vi "StatusUpdateByModID.vi"(8 "error in (no error)":errorcluster, 10 "Status":string, 11 "Accessors:Module ID":i32) -> (0 "error out":errorcluster)   [LabVIEW 2018, in "SensorPlugins.lvlib"]
uses:
  SensorPlugins.lvlib
  SensorShared/clEventType.ctl
  SensorShared/SensorShared.lvlib
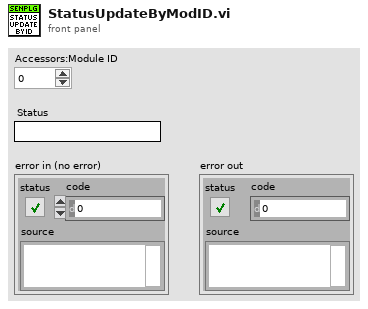
[diagram p1: front panel]
types:
  T1 = typedef "SensorShared.lvlib/clEventType.ctl" = cluster{"ModuleID":i32, "Data":variant}
  T2 = typedef "SensorShared.lvlib/clBroadcastEvents.ctl" = cluster{"DidInit":refnum<user-event>, "StatusUpdate":refnum<user-event>, "ErrorReport":refnum<user-event>, "DidStop":refnum<user-event>, "PathToINI":refnum<user-event>, "SensorReport":refnum<user-event>, "SensorConfig":refnum<user-event>}
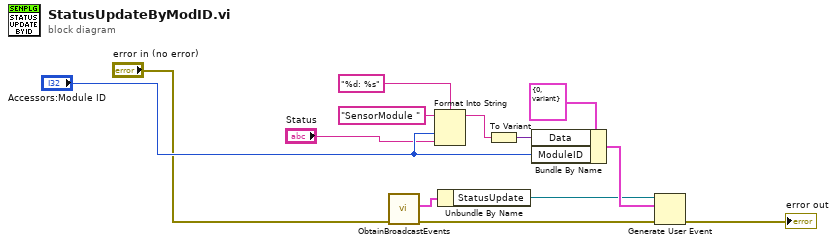
[diagram p0: block diagram]
diagram:
  n1 = call "ObtainBroadcastEvents.vi"("error in (no error)"="error in (no error)") -> ("error out"=w11:errorcluster, "clBroadcastEvents"=w1:T2)  [unwired: 9 in]
  n2 = Format Into String(format string="%d: %s", initial string="SensorModule ", "Accessors:Module ID", "Status") -> (resulting string=w8:string)  [unwired: 1 in, 1 out]
  n3 = Unbundle By Name(w1) -> ("StatusUpdate"=w2:refnum<user-event>)
  n4 = To Variant(anything=w8) -> (Variant=w10:variant)
  n5 = Bundle By Name(cluster=T1 {"ModuleID"=0, "Data"=variant} ("clBroadcast"), "Data"=w10, "ModuleID"="Accessors:Module ID") -> (w4:T1)
  n6 = Generate User Event(user event=w2, event data cluster=w4, error in=w11) -> (error out=→"error out":errorcluster)  [unwired: 1 in, 1 out]
